vi "Remove_NaN_for_ploting.vi"(2 "Array 2":dbl[](array[numeric]) format="%.2f", 3 "Array 1":dbl[](array[numeric]) format="%.2f") -> (0 "Array 2 Out":dbl[](array[numeric]) format="%.2f", 1 "Array 1 Out":dbl[](array[numeric]) format="%.2f")   [LabVIEW 2010]
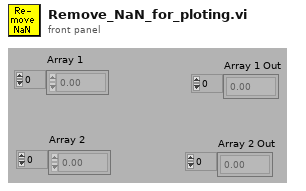
[diagram p1: front panel]
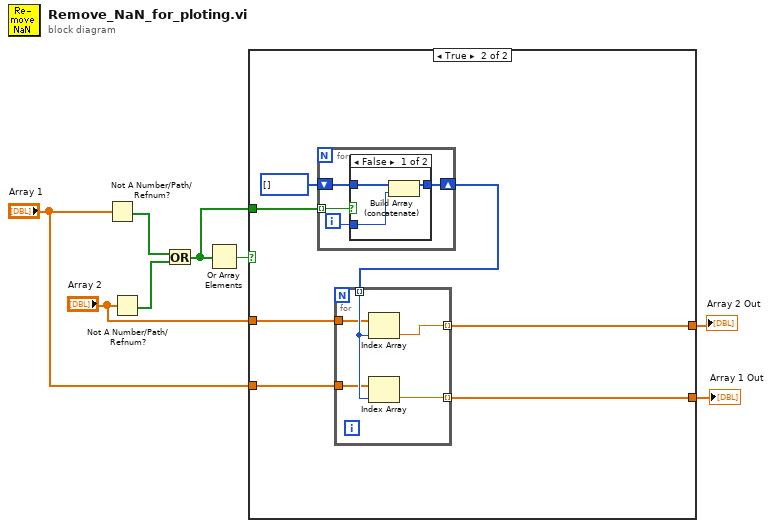
[diagram p0: block diagram]
diagram:
  n1 = Not A Number/Path/Refnum?(number/path/refnum="Array 1") -> (NaN/Path/Refnum?=w7:bool[])
  n2 = Not A Number/Path/Refnum?(number/path/refnum="Array 2") -> (NaN/Path/Refnum?=w8:bool[])
  n3 = Or(x=w7, y=w8) -> (x .or. y?=w5:bool[])
  n4 = Or Array Elements(Boolean array=w5) -> (logical OR=w6:bool)
  n5 = case shown="True" w6 {
    tunnel: w5 -> [_ w16]
    tunnel: "Array 1" -> [w9 w14]
    tunnel: "Array 2" -> [w10 w13]
    tunnel: [w9 w12] -> w2
    tunnel: [w10 w11] -> w1
    frame False {
    }
    frame True {
      n6 = for {
        shift-right: [w24] -> w15
        shift-left: i32[] [] -> [w25]
        tunnel: w16 -> [w23] mode=indexing
        i -> [w26]
        n7 = case shown="False" w23 {
          tunnel: w26 -> [w29 _]
          tunnel: w25 -> [w28 w30]
          tunnel: [w27 w30] -> w24
          frame False {
            n8 = Build Array (concatenate)(w28, w29) -> (w27:i32[])
          }
          frame True {
          }
        }
      }
      n9 = for {
        tunnel: w15 -> [w22] mode=indexing
        tunnel: w14 -> [w21]
        tunnel: w13 -> [w20]
        tunnel: [w19] -> w11 mode=indexing
        tunnel: [w18] -> w12 mode=indexing
        n10 = Index Array(array=w20, index=w22) -> (element=w19:dbl)
        n11 = Index Array(array=w21, index=w22) -> (element=w18:dbl)
      }
    }
  }
  "Array 1 Out" <- w2
  "Array 2 Out" <- w1
